vi "Read PluginINIFilePath.vi"(8 "error in (no error)":errorcluster, 11 "NISTPluginsBase in":refnum<class "MyPluginsBase.lvclass">) -> (0 "error out":errorcluster, 2 "PluginINIFilePath":path, 3 "NISTPluginsBase out":refnum<class "MyPluginsBase.lvclass">)   [LabVIEW 2014]
uses:
  MyPluginsBase.lvclass
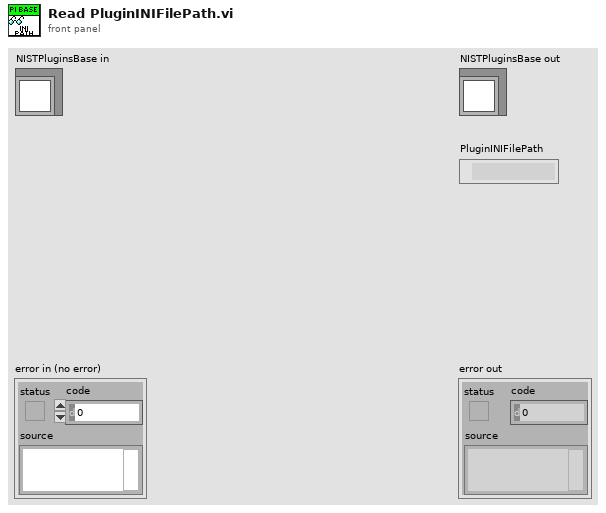
[diagram p1: front panel]
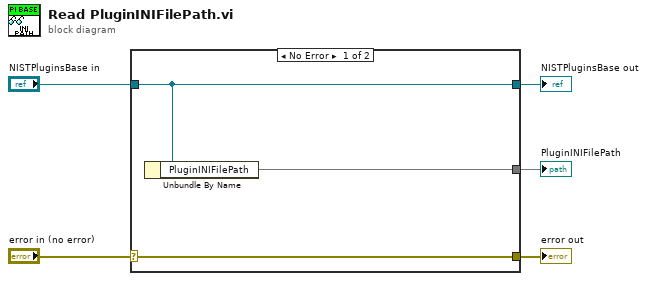
[diagram p0: block diagram]
diagram:
  n1 = case shown="No Error" "error in (no error)" {
    selector: "error in (no error)" -> [w8 w9]
    tunnel: [w8 w9] -> w4
    tunnel: [w7 w10] -> w2
    tunnel: "NISTPluginsBase in" -> [w7 w10]
    tunnel: [w6 _] -> w1
    frame No Error {
      n2 = Unbundle By Name(w7) -> ("PluginINIFilePath"=w6)
    }
    frame Error {
    }
  }
  "error out" <- w4
  "NISTPluginsBase out" <- w2
  "PluginINIFilePath" <- w1
